vi "Sequence.Prod.LoadImg.vi"(9 "corners":cluster{"X":i32, "Y":i32}[](array[cluster]), 10 "path":path) -> (2 "img":picture)   [LabVIEW 2016]
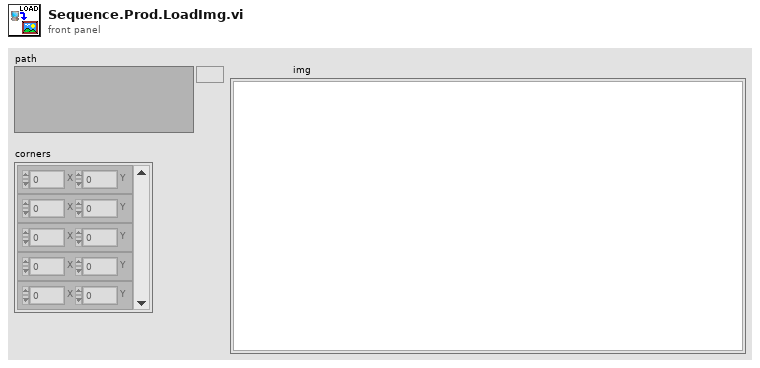
[diagram p1: front panel]
types:
  T1 = typedef "imagedata.ctl" = cluster{"image type":i32, "image depth":i32, "image":u8[], "mask":u8[], "colors":u32[], "Rectangle":cluster{"left":i16, "top":i16, "right":i16, "bottom":i16}}
  T2 = cluster{"left":i16, "top":i16, "right":i16, "bottom":i16}
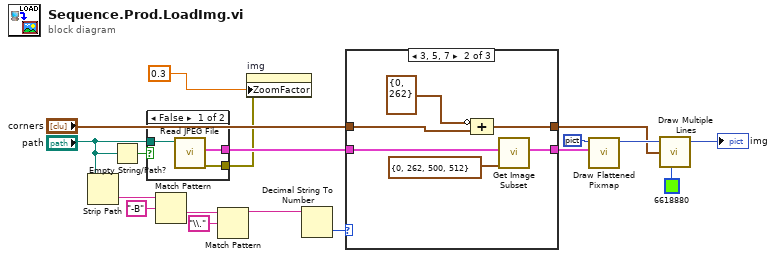
[diagram p0: block diagram]
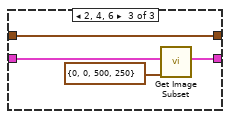
[diagram p3: hidden frame]
diagram:
  n1 = Strip Path(path="path") -> (name=w16:string)  [unwired: 1 out]
  n2 = Empty String/Path?(string/path="path") -> (empty?=w17:bool)
  n3 = case shown="False" w17 {
    tunnel: "path" -> [w21 _]
    tunnel: [w20 _] -> w1
    tunnel: [w19 _] -> w10
    frame False {
      n4 = call <vilib>:"Read JPEG File.vi"("path to JPEG file"=w21) -> ("error out"=w20:errorcluster, "image data"=w19:T1)  [unwired: 8 in, 1 out]
    }
    frame True {
    }
  }
  n5 = Match Pattern(string=w16, regular expression="-B") -> (after substring=w14:string)  [unwired: 1 in, 3 out]
  n6 = Match Pattern(string=w14, regular expression="\\.") -> (before substring=w12:string)  [unwired: 1 in, 3 out]
  n7 = property on="img" class="Pict"(error in=w1, "ZoomFactor"=0.3) -> ()  [unwired: 1 in, 2 out]
  n8 = Decimal String To Number(string=w12) -> (number=w11:i32)  [unwired: 2 in, 1 out]
  n9 = case shown="3, 5, 7" w11 {
    tunnel: w10 -> [w23 w29 w33]
    tunnel: [w23 w28 w31] -> w9
    tunnel: "corners" -> [w22 w25 w30]
    tunnel: [w22 w26 w30] -> w5
    frame Default {
    }
    frame 3, 5, 7 {
      n10 = Compound Arithmetic op=ADD(invert cluster{"X":i32, "Y":i32} {"X"=0, "Y"=262} ("pos"), w25) -> (w26:cluster{"X":i32, "Y":i32}[])
      n11 = call <vilib>:"Get Image Subset.vi"("subset rect"=T2 {"left"=0, "top"=262, "right"=500, "bottom"=512}, "image data"=w29) -> ("image subset"=w28:T1)  [unwired: 4 in, 1 out]
    }
    frame 2, 4, 6 {
      n12 = call <vilib>:"Get Image Subset.vi"("subset rect"=T2 {"left"=0, "top"=0, "right"=500, "bottom"=250}, "image data"=w33) -> ("image subset"=w31:T1)  [unwired: 4 in, 1 out]
    }
  }
  n13 = call <vilib>:"Draw Flattened Pixmap.vi"("image data"=w9, "picture"=picture data[5B]) -> ("new picture"=w7:picture)  [unwired: 7 in]
  n14 = call <vilib>:"Draw Multiple Lines.vi"("picture"=w7, "line endpoints"=w5, "color(black)"=u32 6618880) -> ("new picture"=→"img":picture)  [unwired: 6 in]
